vi "DB UI - Calibration History.vi"(7 "DB Connection":T3={"Open"=TRUE, "Close"=TRUE}, 8 "error in (no error)":errorcluster, 9 "EquipmentID Description":string, 10 "[EquipmentId]":string caption="Equipment ID", 11 "connection reference":T1) -> (0 "SUMMARY":errorcluster, 3 "connection reference 2":T1)   [LabVIEW 2013]
uses:
  <vilib>/addons/database/Connection.llb/Conn ObjectReference.ctl
  Controls/DB - OpenClose.ctl
  <vilib>/Utility/miscctls.llb/LVPointTypeDef.ctl
  <vilib>/addons/database/Connection.llb/Conn Execute.vi
  <vilib>/addons/database/Recordset.llb/Rec Fetch Recordset Data (R).vi
  <vilib>/addons/database/Recordset.llb/Rec Destroy - Connection.vi
  Controls/Global SRTRS.vi
  <vilib>/addons/database/Connection.llb/DB Tools Open Connec (String).vi
  <vilib>/addons/database/_DB Variant To Data/Database Variant To Data.xnode
  <vilib>/addons/database/NI_Database_API.lvlib
panel:
  in  "Tab Control":enum32{"Debug"}(tab)
  in  "DB.Schema.Table\nAdmin.EquipCalibHistory":string="SRTRS.Admin.EquipCalibHistory"
  out "SQL Statement":string
  out "Connection Information":T2={"Connection "="SQL Server 32bit HPEnvy", "Username"="admin", "Password"="admin123"}
  out "Close 2":errorcluster
  in  "CellBG New Cells":u32(colorbox)=16777225
  in  "CellBG Unused Cells":u32(colorbox)=16777238
  in  "CellBG ColHdrs":u32(colorbox)=11776947
  in  "Equipment ID Header [CaptionOnly]":string caption="Header"
  in  "Report List":i32(listbox)=-1 caption="List"
  in  "Close":bool caption="Setup Save"
  # "2014-10-28 13:44\nh.[PlantId]                          ,p.[Description]           ,h.[StationId]                  ,st.[Description]             ,sy.[SystemId]                ,sy.[Description]           ,h.[LastSavedBy]           ,h.[LastSavedOn]          ,t.[PerformedOn]"
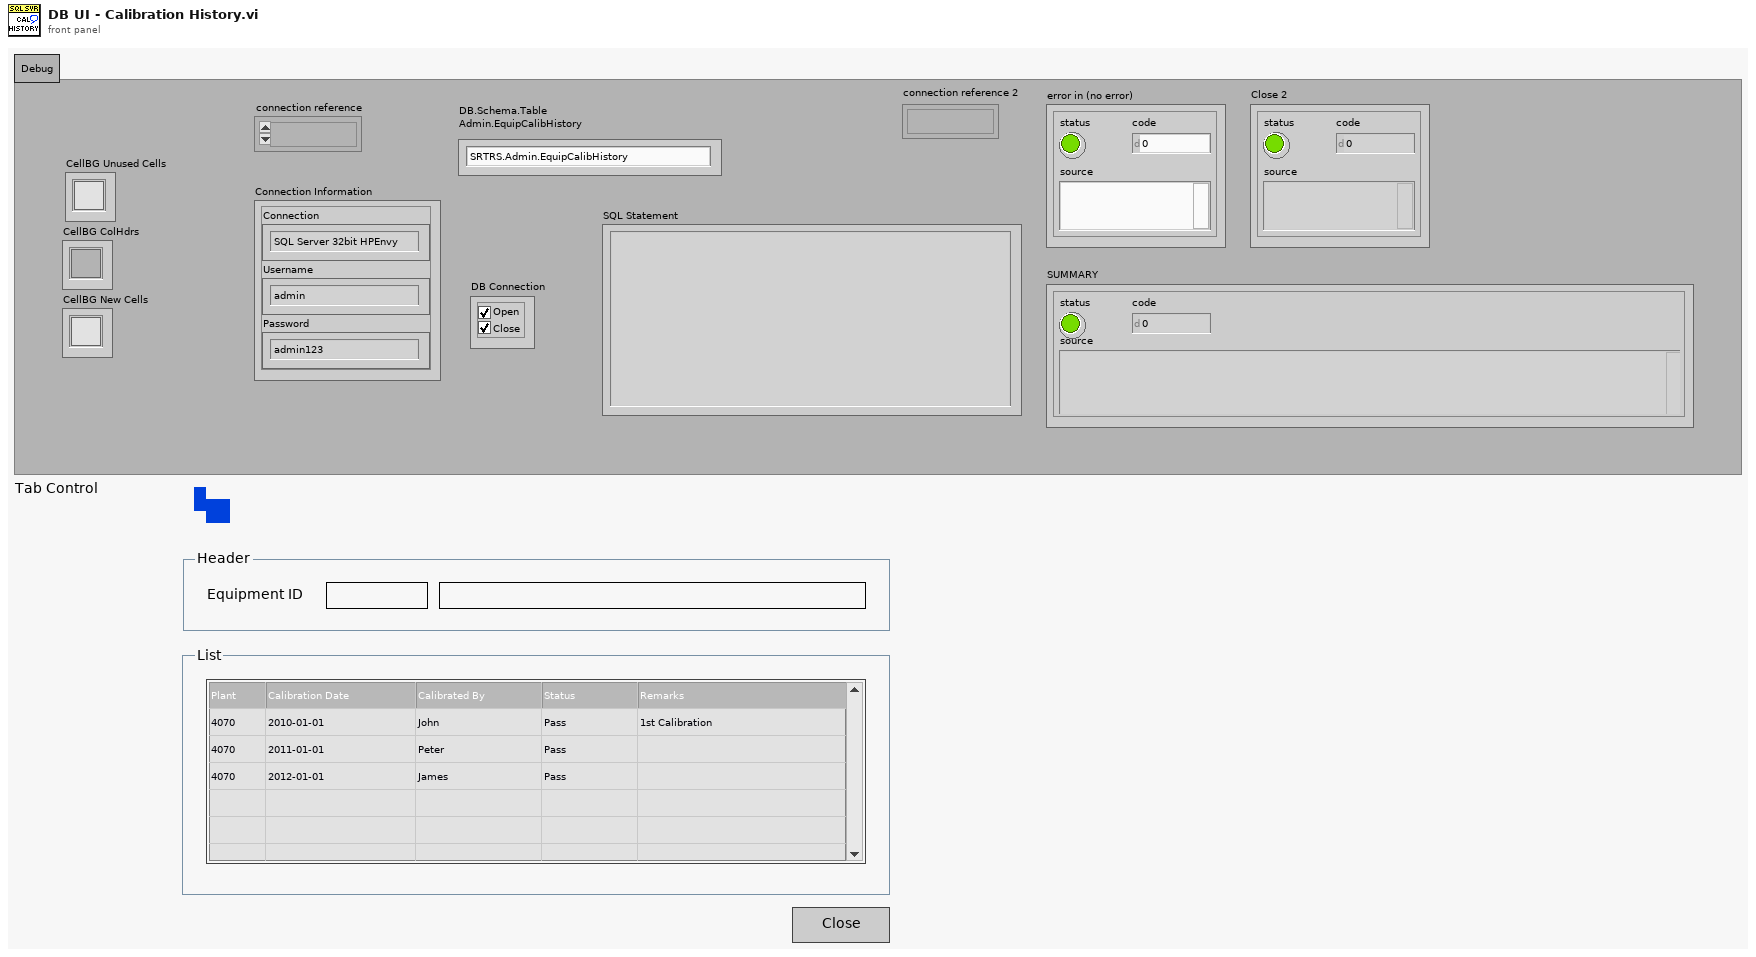
[diagram p1: front panel]
types:
  T1 = typedef "NI_Database_API.lvlib/Conn ObjectReference.ctl" = refnum<k1>
  T2 = cluster{"Connection ":string, "Username":string, "Password":string}
  T3 = typedef "DB - OpenClose.ctl" = cluster{"Open":bool, "Close":bool}
  T4 = typedef "LVPointTypeDef.ctl" = cluster{"Horizontal":i16, "Vertical":i16}
  T5 = typedef "Enum - InteractiveMode-SubVIMode.ctl" = enum16{"Interactive", "subVI Mode"}
  T6 = typedef "DB - DB.Schema.Table.ctl" = cluster{"DB":string, "Schema":string, "Table":string}
  T7 = typedef "Connection Information Cluster.ctl" = cluster{"Connection ":string, "Username":string, "Password":string}
  T8 = typedef "NI_Database_API.lvlib/Rec ObjectReference.ctl" = refnum<k1>
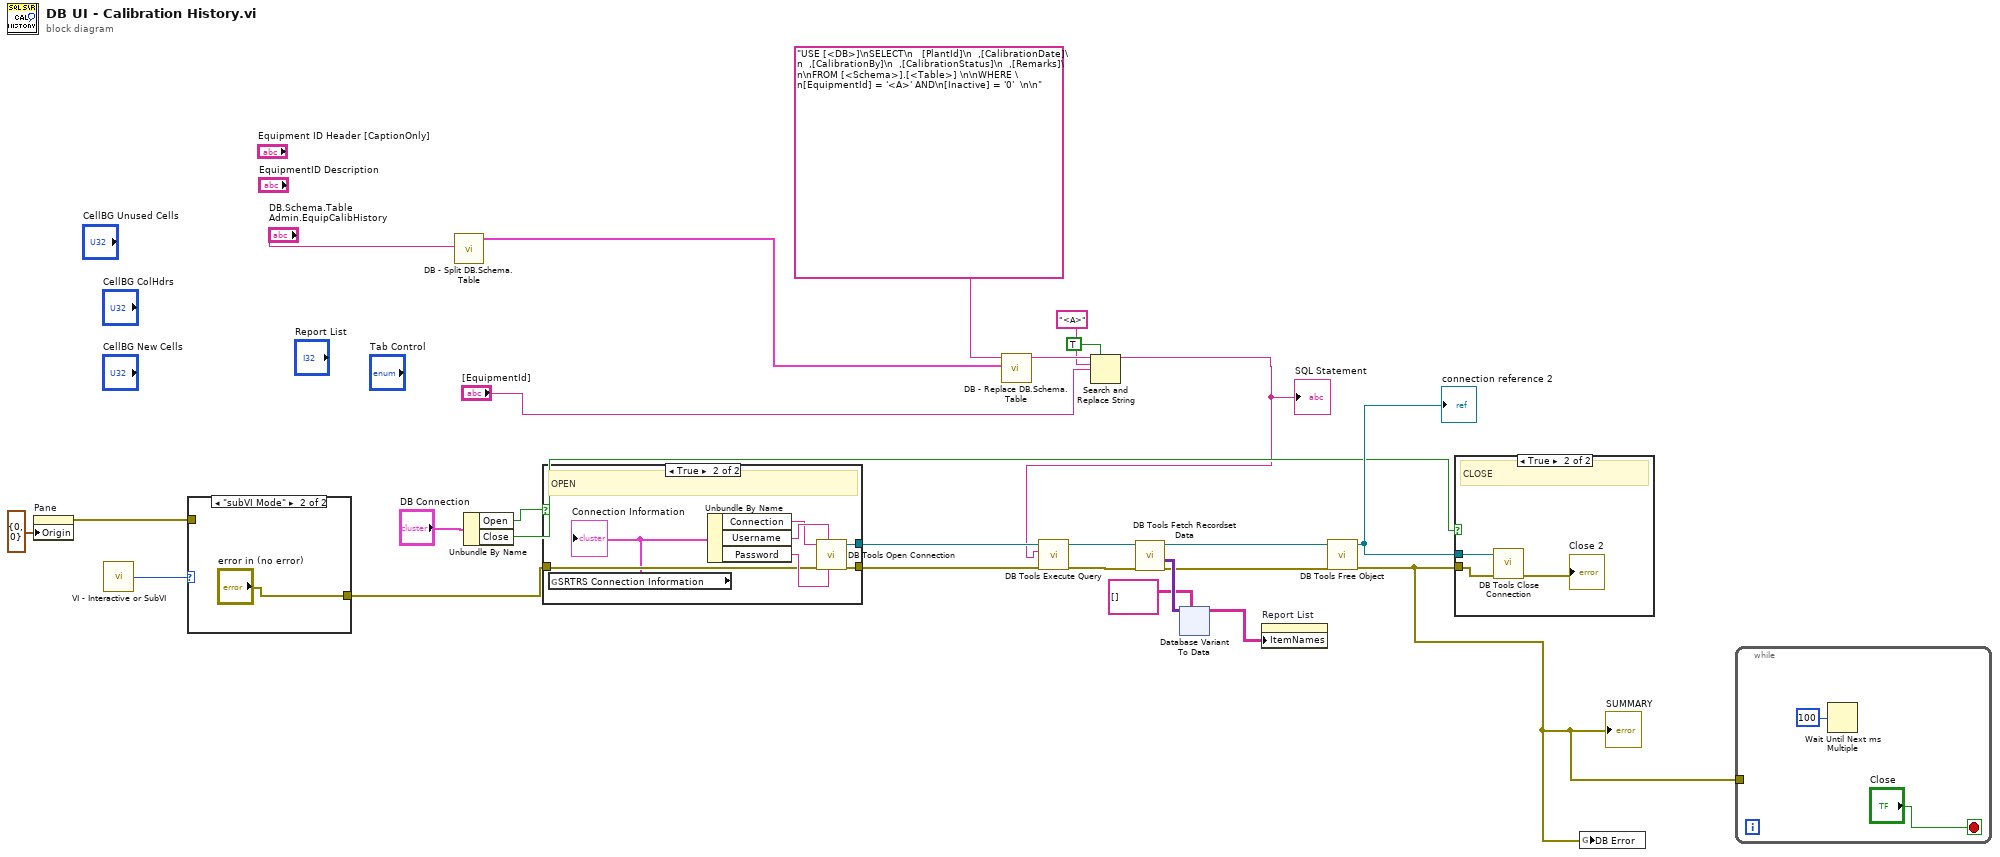
[diagram p0: block diagram]
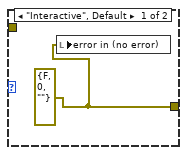
[diagram p3: hidden frame]
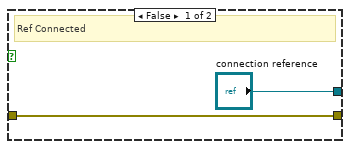
[diagram p4: hidden frame]
diagram:
  n1 = property on="Pane" class="Pane"("Origin"=T4 {"Horizontal"=0, "Vertical"=0}) -> (error out=w5:errorcluster)  [unwired: 2 in, 1 out]
  n2 = call "VI - Interactive or SubVI.vi"() -> ("Mode"=w24:T5)  [unwired: 5 in]
  n3 = case shown="\"subVI Mode\"" w24 {
    tunnel: [w27 "error in (no error)"] -> w23
    tunnel: w5 -> [_ _]
    frame "Interactive", Default {
      w27 = errorcluster {"status"=FALSE, "code"=0, "source"=""} ("error in (no error)")
      n4 = local write "error in (no error)"(w27) -> ()
    }
    frame "subVI Mode" {
    }
  }
  n5 = call "DB - Split DB.Schema.Table.vi"("DB.Schema.Table"="DB.Schema.Table\nAdmin.EquipCalibHistory") -> ("DB.Schema.Table"=w11:T6)  [unwired: 10 in]
  n6 = Unbundle By Name("DB Connection") -> ("Open"=w25:bool, "Close"=w13:bool)
  n7 = case shown="True" w25 {
    tunnel: ["connection reference" w34] -> w16
    tunnel: w23 -> [w29 w33]
    tunnel: [w29 w32] -> w15
    frame False {
      # "Ref Connected"
    }
    frame True {
      # "OPEN"
      n8 = global read "Global SRTRS.vi" "SRTRS Connection Information"() -> (w31:T7)
      "Connection Information" <- w31
      n9 = Unbundle By Name(w31) -> ("Connection"=w36:string, "Username"=w37:string, "Password"=w35:string)
      n10 = call-poly <vilib>:"DB Tools Open Connection.vi"("password"=w35, "userID"=w37, "error in (no error)"=w33, "connection information"=w36) -> ("error out"=w32:errorcluster, "connection reference"=w34:T1)  [unwired: 4 in]
    }
  }
  n11 = call "DB - Replace DB.Schema.Table.vi"("DB.Schema.Table"=w11, "string in"="USE [<DB>]\nSELECT\n   [PlantId]\n  ,[CalibrationDate]\n  ,[CalibrationBy]\n  ,[CalibrationStatus]\n  ,[Remarks]\n\nFROM [<Schema>].[<Table>] \n\nWHERE \n[EquipmentId] = '<A>' AND\n[Inactive] = '0'  \n\n") -> ("string out"=w9:string)  [unwired: 8 in, 1 out]
  n12 = Search and Replace String(replace all?=TRUE ("replace all? (F)"), input string=w9, search string="<A>", replace string="[EquipmentId]") -> (result string=w2:string)  [unwired: 4 in, 3 out]
  "SQL Statement" <- w2
  n13 = call-poly <vilib>:"DB Tools Execute Query.vi"("error in (no error)"=w15, "SQL query"=w2, "connection reference"=w16) -> ("error out"=w22:errorcluster, "recordset reference"=w21:T8)  [unwired: 5 in]
  n14 = call-poly <vilib>:"DB Tools Fetch Recordset Data.vi"("error in (no error)"=w22, "recordset reference"=w21) -> ("error out"=w17:errorcluster, "recordset data"=w20:variant[][], "recordset reference out"=w18:T8)  [unwired: 3 in]
  n15 = xnode "Database Variant To Data"("database variant"=w20, "type"=string[][] []) -> ("data"=w1:string[][])  [unwired: 1 in, 1 out]
  n16 = property on="Report List" class="MCListbox (strict)"("ItemNames"=w1) -> ()  [unwired: 2 in, 2 out]
  n17 = call-poly <vilib>:"DB Tools Free Object.vi"("error in (no error)"=w17, "recordset reference"=w18) -> ("error out"=w3:errorcluster, "connection reference"=w14:T1)  [unwired: 8 in]
  "SUMMARY" <- w3
  "connection reference 2" <- w14
  n18 = case shown="True" w13 {
    tunnel: w14 -> [_ w40]
    tunnel: w3 -> [_ w39]
    frame False {
      # "Ref Connected"
    }
    frame True {
      # "CLOSE"
      n19 = call <vilib>:"DB Tools Close Connection.vi"("error in (no error)"=w39, "connection reference"=w40) -> ("error out"=→"Close 2":errorcluster)  [unwired: 5 in]
    }
  }
  n20 = global write "Global SRTRS.vi" "DB Error"(w3) -> ()
  n21 = while {
    tunnel: w3 -> [_]
    stop <- "Close" stop-if-true
    n22 = Wait Until Next ms Multiple(millisecond multiple=u32 100) -> ()  [unwired: 1 out]
  }
